vi "distance_processing.vi"(0 "Trace info in":T4, 2 "Time Stamp":timestamp, 3 "Ref carrier amplitudes":T1 format="%#_3p", 5 "Config":T7={"IO params"={"Conversion"={"Rate"=4.0, "In cards"=2, "Out channels"=4}, "Carriers"={"Phase shift"=180.0, "Levels"=[[0.8, 0.8, 0.8], [0.03, 0.03, 0.03]], "Delay samples"=73.15}}, "High rate STFT"={"Win param"=101.5, "Window type"=61, "Win order"=2, "DFT size"=64, "Channels"=[7], "Oversample"=64}, "Low rate STFT"={"Win param"=120.0, "Window type"=61, "Win order"=8, "DFT size"=64, "Channels"=[7], "Oversample"=64}, "Filtering"={"Hum"={"Frequency"=0.0, "Tc"=0.0, "Limit"=101.5, "FFT filter"=FALSE, "Detrend mode"=enum."Robust linear", "Enable"=FALSE}, "Kalman"={"Process noise"=101.5, "Measure noise"=101.5}, "Distortion"={"LF cut"=101.5, "Tc"=3.0, "Limit"=101.5, "FFT filter"=FALSE, "Detrend mode"=enum."Robust linear", "Enable"=FALSE}}} {"Filtering"."Distortion"."Limit" format="%#_3p"; "Filtering"."Distortion"."LF cut" format="%#_3p"; "Filtering"."Kalman"."Measure noise" format="%#_3p"; "Filtering"."Kalman"."Process noise" format="%#_3p"; "Filtering"."Hum"."Limit" format="%#_3p"; "Filtering"."Hum"."Frequency" format="%#_4p"; "Low rate STFT"."Oversample" min=1 step=1; "Low rate STFT"."Channels" min=0 step=1; "Low rate STFT"."DFT size" min=1 step=1; "Low rate STFT"."Window type" items=["Rectangle"=0, "Hanning"=1, "Hamming"=2, "Blackman-Harris"=3, "Exact Blackman"=4, "Blackman"=5, "Flat Top"=6, "4 Term B-Harris "=7, "7 Term B-Harris"=8, "Low Sidelobe"=9, "Blackman Nuttall"=11, "Triangle"=30, "Bartlett-Hanning"=31, "Bohman"=32, "Parzen"=33, "Welch"=34, "Kaiser"=60, "Dolph-Chebyshev"=61, "Gaussian"=62]; "High rate STFT"."Oversample" min=1 step=1; "High rate STFT"."Channels" min=0 step=1; "High rate STFT"."DFT size" min=1 step=1; "High rate STFT"."Window type" items=["Rectangle"=0, "Hanning"=1, "Hamming"=2, "Blackman-Harris"=3, "Exact Blackman"=4, "Blackman"=5, "Flat Top"=6, "4 Term B-Harris "=7, "7 Term B-Harris"=8, "Low Sidelobe"=9, "Blackman Nuttall"=11, "Triangle"=30, "Bartlett-Hanning"=31, "Bohman"=32, "Parzen"=33, "Welch"=34, "Kaiser"=60, "Dolph-Chebyshev"=61, "Gaussian"=62]; "IO params"."Carriers"."Levels" min=0.0 step=0.1; "IO params"."Conversion"."Rate" format="%#_8g"}, 6 "Carrier amplitudes":T1 format="%#_3p", 10 "Output options":T2={"Source"=enum."X", "Sensor"=enum."X", "Sense"=FALSE, "Distance"=FALSE, "LF corner"=0.1, "RMS Tc"=5.0}, 11 "Modulation info":T15={"Fs full"=0.0, "Fs high"=0.0, "Fs low"=0.0, "Read size"=0, "FFT size low"=5000, "df low"=5000.0, "High carriers"=[], "Low carriers"=[], "Hi channels at low"=[7]} {"Hi channels at low" min=0 step=1; "Low carriers" format="%#_6p"; "High carriers" format="%#_6p"}, 12 "Calibration":T13 {"r bias" format="%_3p"; "Ks" format="%#_3p"}, 13 "Reset":bool, 15 "Reset RMS":bool, 16 "Measurements In":T16 {"RMS" format="%#_3p"; "Relative" format="%.4f"; "Ref distance" format="%.3f"; "DC" format="%.3f"}, 17 "High carrier amplitudes":T14 format="%#_3p") -> (20 "Measurements out":T16 {"RMS" format="%#_3p"; "Relative" format="%.4f"; "Ref distance" format="%.3f"; "DC" format="%.3f"}, 22 "Mean level":dbl[](array[numeric]), 23 "Chart display":waveform(dbl)[](array[waveform]), 26 "Trace info out":T4)   [LabVIEW 2014]
uses:
  measurements.ctl
  modulation_info.ctl
  high_carrier_amplitudes.ctl
  calibration.ctl
  ilemt_config.ctl
  IO_params.ctl
  stft_params.ctl
  <vilib>/Analysis/4window.llb/windowTd.ctl
  filter_params.ctl
  detrend_mode.ctl
  carrier_amplitudes.ctl
  trace_info.ctl
  trace_channel.ctl
  ilemt_status.ctl
  output_options.ctl
  coupling_selector.ctl
  <vilib>/Analysis/NI_AALPro.lvlib
panel:
  # "This is an input (as well as an output) because this is where we keep the reference distance."
  # "This is used by the builtin 1DOF calibration"
  # "High rate time samples of high carrier amplitudes"
  # "Low rate measurement of all carrier amplitudes"
  # "Carrier amplitudes at the time of \"Set ref\""
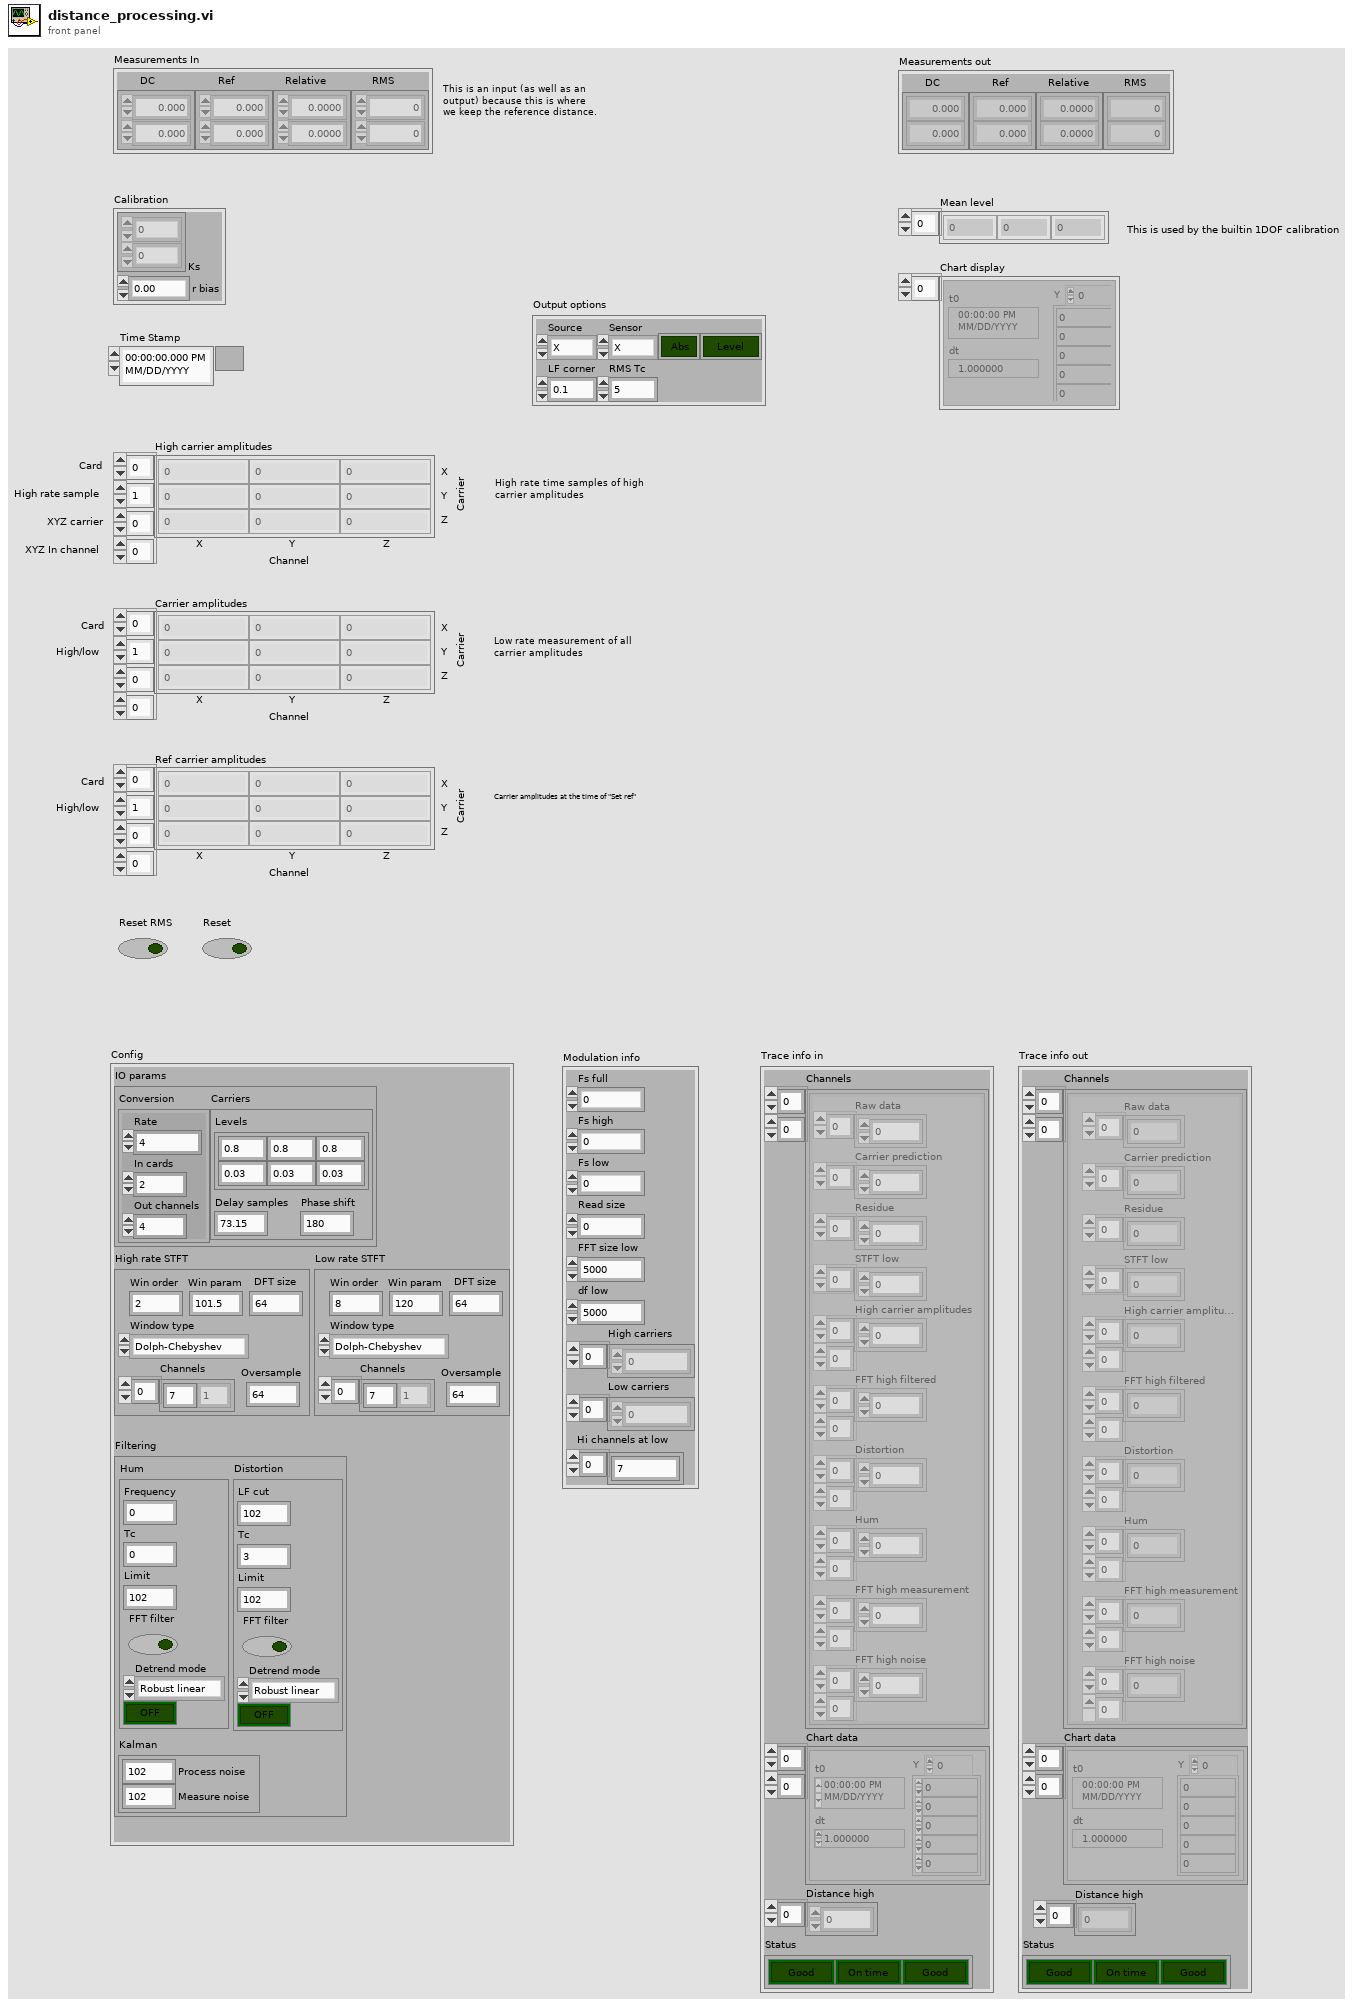
[diagram p1: front panel]
types:
  T1 = typedef "carrier_amplitudes.ctl" = cdb[][][][]
  T2 = typedef "output_options.ctl" = cluster{"Source":T3, "Sensor":T3, "Sense":bool, "Distance":bool, "LF corner":dbl, "RMS Tc":dbl}
  T3 = typedef "coupling_selector.ctl" = enum16{"X", "Y", "Z", "Vector"}
  T4 = typedef "trace_info.ctl" = cluster{"Channels":T5[][], "Chart data":waveform(dbl)[][], "Distance high":dbl[], "Status":T6}
  T5 = typedef "trace_channel.ctl" = cluster{"Raw data":dbl[], "Carrier prediction":dbl[], "Residue":dbl[], "STFT low":cdb[], "High carrier amplitudes":cdb[][], "FFT high filtered":cdb[][], "Distortion":cdb[][], "Hum":cdb[][], "FFT high measurement":cdb[][], "FFT high noise":dbl[][]}
  T6 = typedef "ilemt_status.ctl" = cluster{"NaN":bool, "Backlog":bool, "Clipping":bool}
  T7 = typedef "ilemt_config.ctl" = cluster{"IO params":T8, "High rate STFT":T9, "Low rate STFT":T9, "Filtering":T11}
  T8 = typedef "IO_params.ctl" = cluster{"Conversion":cluster{"Rate":dbl, "In cards":u32, "Out channels":u32}, "Carriers":cluster{"Phase shift":dbl, "Levels":dbl[][], "Delay samples":dbl}}
  T9 = typedef "stft_params.ctl" = cluster{"Win param":dbl, "Window type":T10, "Win order":i32, "DFT size":i32, "Channels":i32[], "Oversample":i32}
  T10 = typedef "NI_AALPro.lvlib/windowTd.ctl" = u32
  T11 = typedef "filter_params.ctl" = cluster{"Hum":cluster{"Frequency":dbl, "Tc":dbl, "Limit":dbl, "FFT filter":bool, "Detrend mode":T12, "Enable":bool}, "Kalman":cluster{"Process noise":dbl, "Measure noise":dbl}, "Distortion":cluster{"LF cut":dbl, "Tc":dbl, "Limit":dbl, "FFT filter":bool, "Detrend mode":T12, "Enable":bool}}
  T12 = typedef "detrend_mode.ctl" = enum16{"Zero mean", "Linear", "Robust linear"}
  T13 = typedef "calibration.ctl" = cluster{"Ks":dbl[], "r bias":dbl}
  T14 = typedef "high_carrier_amplitudes.ctl" = cdb[][][][]
  T15 = typedef "modulation_info.ctl" = cluster{"Fs full":dbl, "Fs high":dbl, "Fs low":dbl, "Read size":i32, "FFT size low":i32, "df low":dbl, "High carriers":dbl[], "Low carriers":dbl[], "Hi channels at low":i32[]}
  T16 = typedef "measurements.ctl" = cluster{"DC":dbl[], "Ref distance":dbl[], "Relative":dbl[], "RMS":dbl[]}
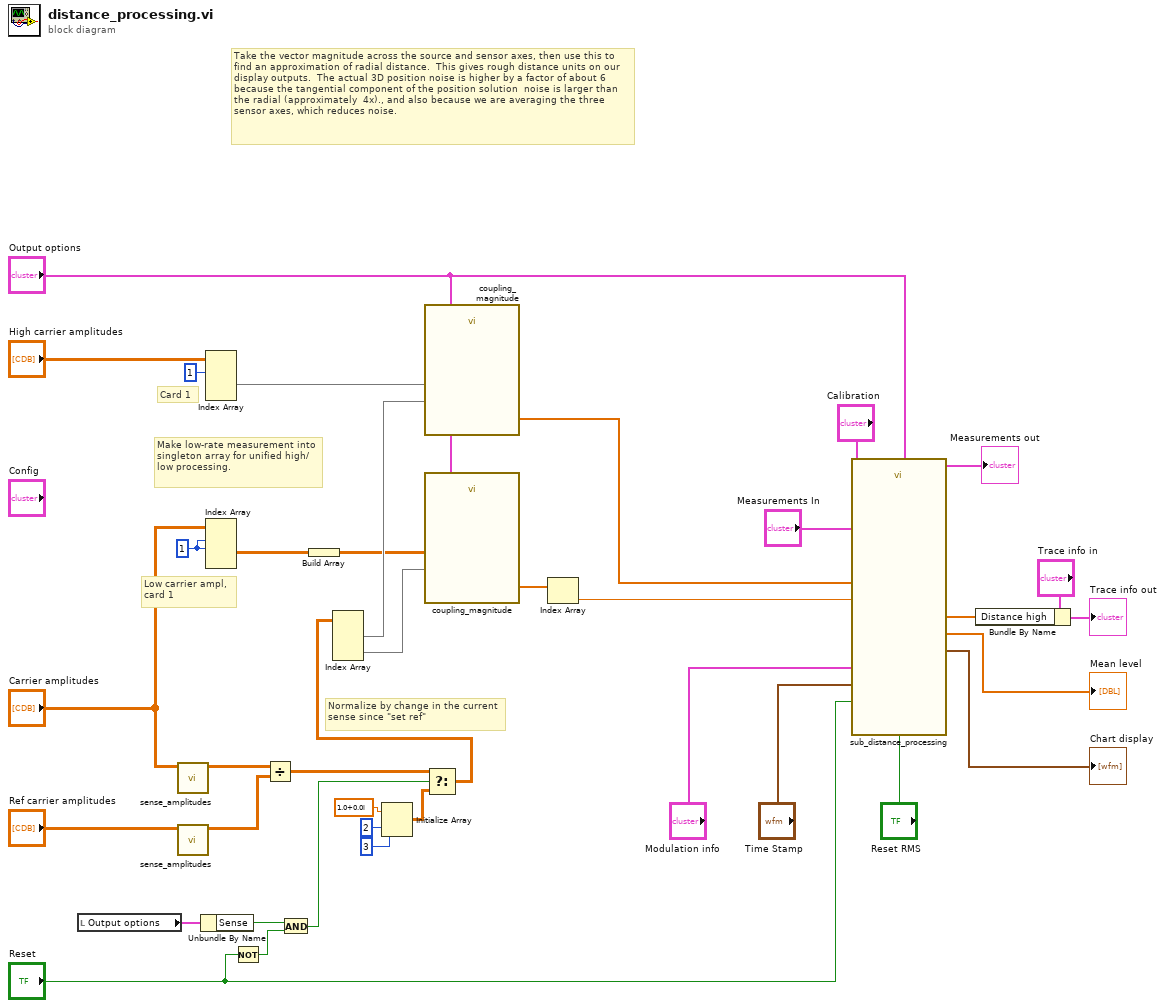
[diagram p0: block diagram]
diagram:
  w12 = 1 ("disabled index (row)")
  # "Make low-rate measurement into singleton array for unified high/low processing."
  # "Take the vector magnitude across the source and sensor axes, then use this to find an approximation of radial distance.  This gives rough distance units on our display outputs.  The actual 3D position noise is higher by a factor of about 6 because the tangential component of the position solution  noise is larger than the radial (approximately  4x)., and also because we are averaging the three sensor axes, which reduces noise."
  # "Card 1"
  # "Normalize by change in the current sense since \"set ref\""
  # "Low carrier ampl,\ncard 1"
  n1 = local read "Output options"() -> (w2:T2)
  n2 = call "sense_amplitudes.vi"("Ref carrier amplitudes in"="Carrier amplitudes") -> ("Sense amplitudes"=w13:cdb[][])  [unwired: 10 in]
  n3 = call "sense_amplitudes.vi"("Ref carrier amplitudes in"="Ref carrier amplitudes") -> ("Sense amplitudes"=w24:cdb[][])  [unwired: 10 in]
  n4 = Unbundle By Name(w2) -> ("Sense"=w17:bool)
  n5 = Index Array(array="High carrier amplitudes", index (dim 0)=1 ("index (vol)")) -> (element=w9:cdb[][][])  [unwired: 3 in]
  n6 = Index Array(array="Carrier amplitudes", index (dim 0)=w12, index (dim 1)=w12) -> (element=w4:cdb[][])  [unwired: 2 in]
  n7 = Not(x="Reset") -> (.not. x?=w18:bool)
  n8 = Divide(x=w13, y=w24) -> (x/y=w23:cdb[][])
  n9 = And(x=w17, y=w18) -> (x .and. y?=w16:bool)
  n10 = Build Array(w4) -> (w3:cdb[][][])
  n11 = Initialize Array(cdb 1.0+0.0i, 2 ("dimension size"), 3 ("dimension size")) -> (w19:cdb[][])
  n12 = Select(t=w23, s=w16, f=w19) -> (s? t:f=w27:cdb[][])
  n13 = Index Array(array=w27) -> (element #1=w29:cdb[], element #2=w7:cdb[])  [unwired: 4 in]
  n14 = call "coupling_magnitude.vi"("Carrier sense"=w29, "Carrier amplitudes"=w9, "Output options"="Output options") -> ("Magnitudes"=w25:dbl[])  [unwired: 8 in]
  n15 = call "coupling_magnitude.vi"("Carrier sense"=w7, "Carrier amplitudes"=w3, "Output options"="Output options") -> ("Magnitudes"=w6:dbl[])  [unwired: 8 in]
  n16 = Index Array(array=w6) -> (element=w5:dbl)  [unwired: 1 in]
  n17 = call "sub_distance_processing.vi"("Magnitude high"=w25, "Calibration"="Calibration", "Measurements In"="Measurements In", "Magnitude low"=w5, "Modulation info"="Modulation info", "Reset"="Reset", "Output options"="Output options", "Reset RMS"="Reset RMS", "Time Stamp"="Time Stamp") -> ("Measurements out"=→"Measurements out":T16, "Mean level"=→"Mean level":dbl[], "Chart display"=→"Chart display":waveform(dbl)[], "Distance high"=w32:dbl[])  [unwired: 3 in]
  n18 = Bundle By Name(cluster="Trace info in", "Distance high"=w32) -> (→"Trace info out":T4)
